vi "BentStyle_Create.vi"(5 "error in (no error)":errorcluster) -> (14 "reference out":refnum<class "BentStyle.lvclass">, 19 "error out":errorcluster)   [LabVIEW 2020, in "BentStyle.lvclass"]
doc: "Creates and initializes a new BentStyle object.\n\nThis object should be destroyed using a BentStyle destructor VI.\n\n[GOOP 2.1]"
uses:
  <resource>/Framework/Providers/Open_GDS/UML/BentStyle_class/BentStyle.lvclass
  <resource>/Framework/Providers/Open_GDS/UML/BentStyle_class/BentStyleType.ctl
panel:
  in  "BentStyle":T1
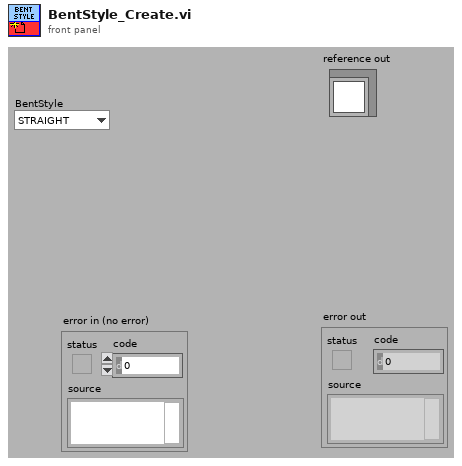
[diagram p1: front panel]
types:
  T1 = typedef "BentStyle.lvclass/BentStyleType.ctl" = enum16{"STRAIGHT", "HV", "VH", "HVH", "VHV", "ARC"}
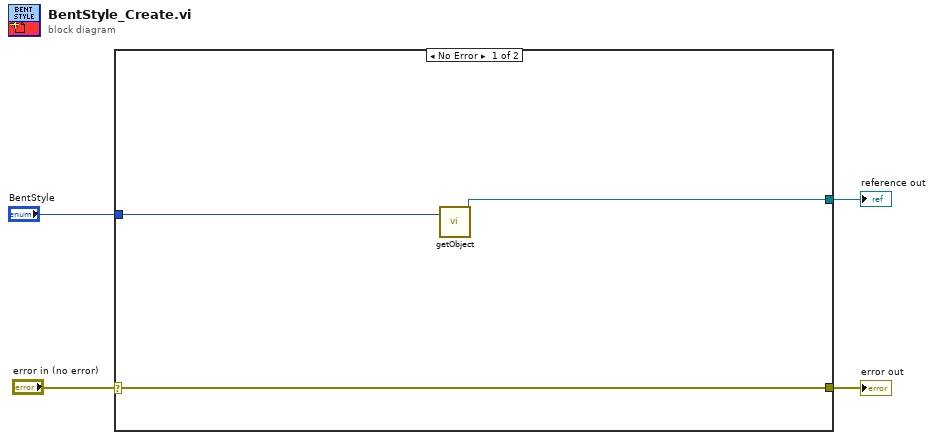
[diagram p0: block diagram]
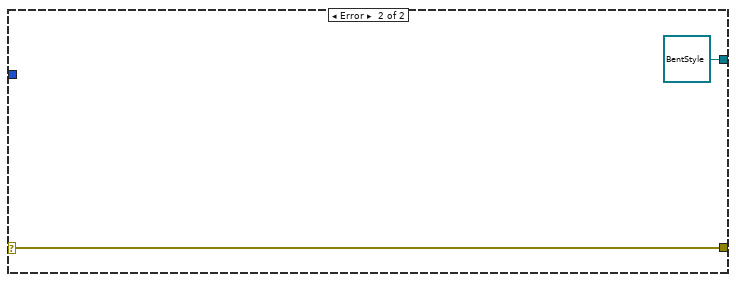
[diagram p2: hidden frame]
diagram:
  n1 = case shown="No Error" "error in (no error)" {
    selector: "error in (no error)" -> [w7 w9]
    tunnel: [w5 refnum<class "BentStyle.lvclass"> refnum ("reference out")] -> w4
    tunnel: [w7 w9] -> w3
    tunnel: "BentStyle" -> [w6 _]
    frame No Error {
      n2 = call <resource>:"getObject.vi"("bentStyle"=w6) -> ("reference out"=w5:refnum<class "BentStyle.lvclass">)  [unwired: 17 in, 1 out]
    }
    frame Error {
    }
  }
  "error out" <- w3
  "reference out" <- w4
